vi "GV-CursorHzoom.vi"(7 "Gviewer in":refnum<class "Gviewer.lvclass">, 8 "error in (no error)":errorcluster, 10 "Pos":cluster{"x":i16, "y":i16}, 11 "pict in":picture) -> (0 "error out":errorcluster, 3 "pict out":picture, 5 "Gviewer out":refnum<class "Gviewer.lvclass">)   [LabVIEW 2020, in "Sgraph_lib_V1.lvlib" / "Gviewer.lvclass"]
doc: "Andre Koelewijn, 14 feb 2021\n\nTime scroll zoom cursor draw"
uses:
  Gviewer.lvclass
  Gviewer.lvclass/Gviewer.ctl
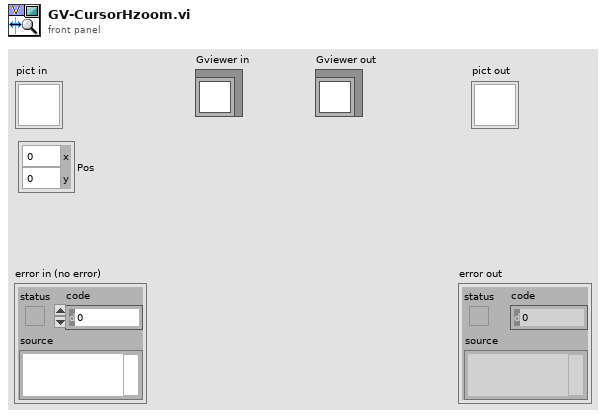
[diagram p1: front panel]
types:
  T1 = cluster{"horizontal":enum16{"left", "center", "right"}, "vertical":enum16{"top", "center", "bottom"}}
  T2 = cluster{"Width":u16, "Style":enum32{"Solid", "Dash", "Dot", "DashDot", "DashDotDot"}}
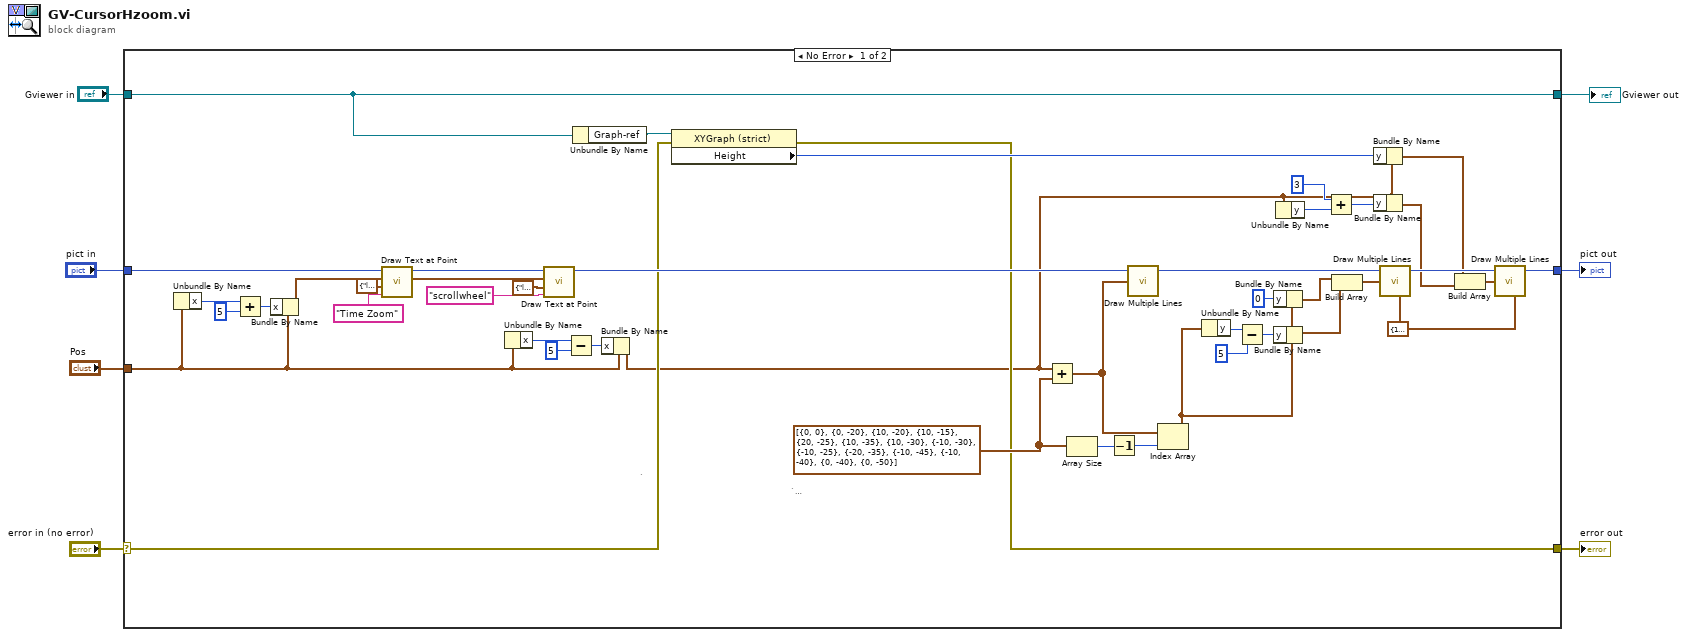
[diagram p0: block diagram]
diagram:
  n1 = case shown="No Error" "error in (no error)" {
    selector: "error in (no error)" -> [w15 w53]
    tunnel: [w16 w53] -> w6
    tunnel: "pict in" -> [w26 w52]
    tunnel: [w35 w52] -> w4
    tunnel: "Pos" -> [w10 _]
    tunnel: "Gviewer in" -> [w8 w51]
    tunnel: [w8 w51] -> w1
    frame No Error {
      w44 = T2 {"Width"=1, "Style"=enum."Dash"} ("pen")
      w49 = cluster{"x":i16, "y":i16}[] [{"x"=0, "y"=0}, {"x"=0, "y"=-20}, {"x"=10, "y"=-20}, {"x"=10, "y"=-15}, {"x"=20, "y"=-25}, {"x"=10, "y"=-35}, {"x"=10, "y"=-30}, {"x"=-10, "y"=-30}, {"x"=-10, "y"=-25}, {"x"=-20, "y"=-35}, {"x"=-10, "y"=-45}, {"x"=-10, "y"=-40}, {"x"=0, "y"=-40}, {"x"=0, "y"=-50}] ("line endpoints")
      # "`"
      # "``"
      n2 = Unbundle By Name(w10) -> ("x"=w11:i16)
      n3 = Add(x=w11, y=i16 5) -> (x+y=w13:i16)
      n4 = Bundle By Name(cluster=w10, "x"=w13) -> (w9:cluster{"x":i16, "y":i16})
      n5 = call <vilib>:"Draw Text at Point.vi"("text"="Time Zoom", "alignment(left, top)"=T1 {"horizontal"=enum."left", "vertical"=enum."bottom"}, "origin"=w9, "picture"=w26) -> ("new picture"=w23:picture)  [unwired: 6 in, 1 out]
      n6 = Unbundle By Name(w10) -> ("x"=w22:i16)
      n7 = call <vilib>:"Draw Text at Point.vi"("text"="scrollwheel", "alignment(left, top)"=T1 {"horizontal"=enum."left", "vertical"=enum."top"}, "origin"=w9, "picture"=w23) -> ("new picture"=w19:picture)  [unwired: 6 in, 1 out]
      n8 = Subtract(x=w22, y=i16 5) -> (x-y=w20:i16)
      n9 = Unbundle By Name(w8) -> ("Graph-ref"=w18:refnum<vi>)
      n10 = Bundle By Name(cluster=w10, "x"=w20) -> (w14:cluster{"x":i16, "y":i16})
      n11 = property class="XYGraph (strict)"(reference=w18, error in=w15) -> (error out=w16:errorcluster, "Height"=w17:u32)  [unwired: 1 out]
      n12 = Add(x=w14, y=w49) -> (x+y=w46:cluster{"x":i16, "y":i16}[])
      n13 = Array Size(array=w49) -> (size(s)=w48:i32)
      n14 = Decrement(x=w48) -> (x-1=w47:i32)
      n15 = call <vilib>:"Draw Multiple Lines.vi"("picture"=w19, "line endpoints"=w46) -> ("new picture"=w50:picture)  [unwired: 7 in]
      n16 = Index Array(array=w46, index=w47) -> (element=w38:cluster{"x":i16, "y":i16})
      n17 = Unbundle By Name(w38) -> ("y"=w43:i16)
      n18 = Subtract(x=w43, y=i16 5) -> (x-y=w41:i16)
      n19 = Bundle By Name(cluster=w38, "y"=i16 0 ("x")) -> (w37:cluster{"x":i16, "y":i16})
      n20 = Bundle By Name(cluster=w38, "y"=w41) -> (w40:cluster{"x":i16, "y":i16})
      n21 = Unbundle By Name(w14) -> ("y"=w34:i16)
      n22 = Add(x=i16 3, y=w34) -> (x+y=w33:i16)
      n23 = Build Array(w37, w40) -> (w45:cluster{"x":i16, "y":i16}[])
      n24 = Bundle By Name(cluster=w14, "y"=w17) -> (w29:cluster{"x":i16, "y":i16})
      n25 = Bundle By Name(cluster=w14, "y"=w33) -> (w30:cluster{"x":i16, "y":i16})
      n26 = call <vilib>:"Draw Multiple Lines.vi"("picture"=w50, "line endpoints"=w45, "pen"=w44) -> ("new picture"=w36:picture)  [unwired: 6 in]
      n27 = Build Array(w29, w30) -> (w31:cluster{"x":i16, "y":i16}[])
      n28 = call <vilib>:"Draw Multiple Lines.vi"("picture"=w36, "line endpoints"=w31, "pen"=w44) -> ("new picture"=w35:picture)  [unwired: 6 in]
    }
    frame Error {
    }
  }
  "error out" <- w6
  "pict out" <- w4
  "Gviewer out" <- w1
